vi "RemNoiseRec.vi"(3 "Data In":i16[][](array[numeric])) -> (1 "Data Out":i16[][](array[numeric]))   [LabVIEW 2022 SP3]
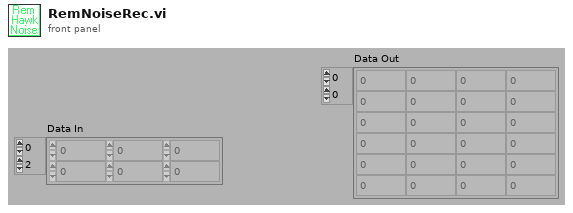
[diagram p1: front panel]
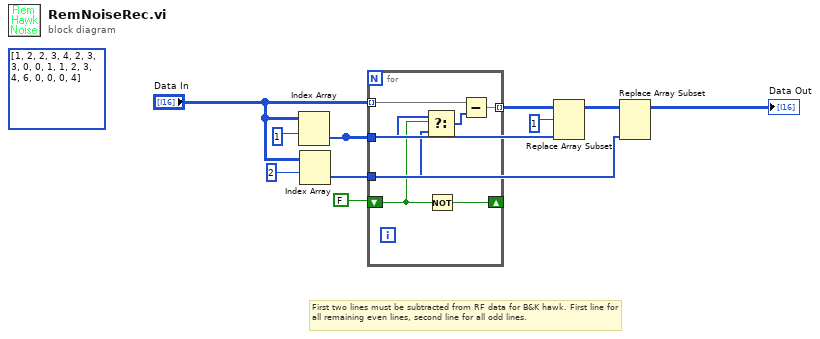
[diagram p0: block diagram]
diagram:
  (unwired) i16[][][] [[[1, 2, 2, 3, 4], [2, 3, 3, 0, 0], [1, 1, 2, 3, 4], [6, 0, 0, 0, 4]]] ("Data")
  # "First two lines must be subtracted from RF data for B&K hawk. First line for all remaining even lines, second line for all odd lines."
  n1 = Index Array(array="Data In", index (row)=1) -> (element=w3:i16[])  [unwired: 1 in]
  n2 = Index Array(array="Data In", index (row)=2) -> (element=w4:i16[])  [unwired: 1 in]
  n3 = for {
    tunnel: "Data In" -> [w14] mode=indexing
    tunnel: w3 -> [w17]
    tunnel: w4 -> [w16]
    tunnel: [w13] -> w6 mode=indexing
    shift-right: [w11] -> _
    shift-left: FALSE -> [w12]
    n4 = Select(t=w17, s=w12, f=w16) -> (s? t:f=w15:i16[])
    n5 = Not(x=w12) -> (.not. x?=w11:bool)
    n6 = Subtract(x=w14, y=w15) -> (x-y=w13:i16[])
  }
  n7 = Replace Array Subset(array=w6, new element=w3, index (row)=1) -> (w5:i16[][])  [unwired: 1 in]
  n8 = Replace Array Subset(array=w5, new element=w4) -> (→"Data Out":i16[][])  [unwired: 2 in]
